vi "Set Safe State.vi"(8 "error in":errorcluster, 9 "timeout (-1)":i32=-1, 11 "Standard Engine Runtime in":refnum<class "synchronous engine runtime.lvclass">) -> (0 "error out":errorcluster, 3 "Standard Engine Runtime out":refnum<class "synchronous engine runtime.lvclass">)   [LabVIEW 2013, in "synchronous engine runtime.lvclass"]
uses:
  synchronous engine runtime.lvclass
  Commands.ctl
  synchronous engine runtime.lvclass/synchronous engine runtime.ctl
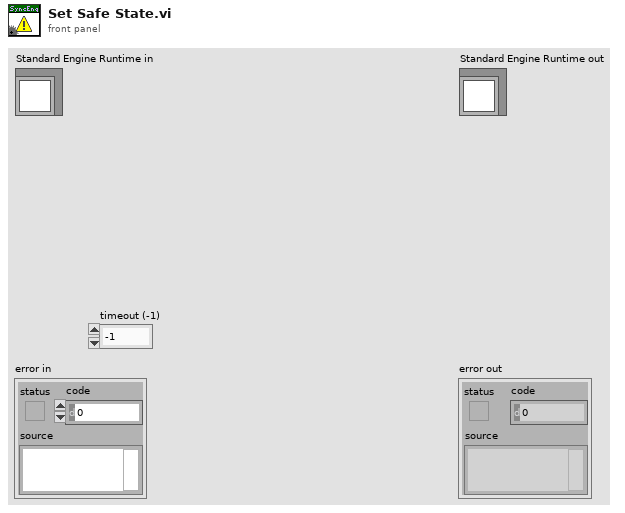
[diagram p1: front panel]
types:
  T1 = typedef "synchronous engine runtime.lvclass/Commands.ctl" = enum16{"Start", "Pause", "Safe State", "Normal", "Stop", "Shutdown"}
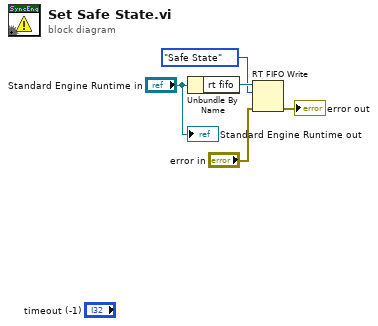
[diagram p0: block diagram]
diagram:
  n1 = Unbundle By Name("Standard Engine Runtime in") -> ("rt fifo"=w4:refnum<k33>)
  n2 = RT FIFO Write(0:w4, 1:Commands."Safe State" ("element"), 3:"error in") -> (11:→"error out":errorcluster)  [unwired: 2 in, 3 out]
  "Standard Engine Runtime out" <- "Standard Engine Runtime in"
